vi "加载界面.vi"() -> ()   [LabVIEW 2019]
panel:
  out "错误输出":errorcluster
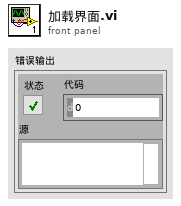
[diagram p1: front panel]
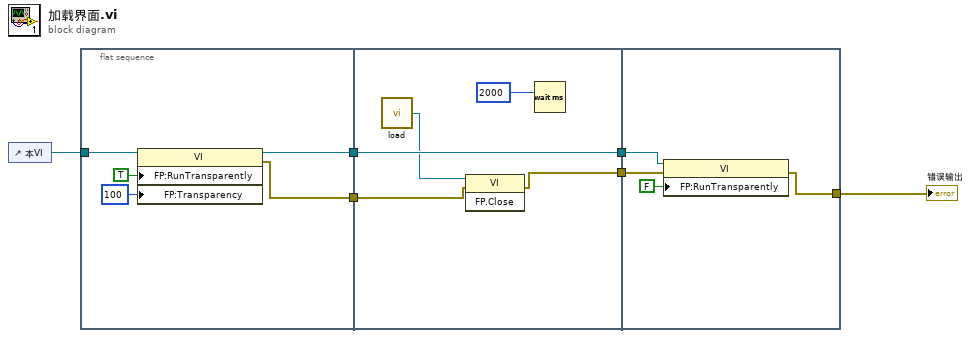
[diagram p0: block diagram]
diagram:
  n1 = control-ref of="本VI"() -> (w6:refnum<vi>)
  n2 = flat-sequence {
    tunnel: w6 -> [w11]
    tunnel: [w8] -> w4
    tunnel: [w7] -> w3
    tunnel: [w15] -> w5
    tunnel: w4 -> [w15]
    tunnel: w3 -> [w14]
    tunnel: [w13] -> w2
    tunnel: w5 -> [w20]
    tunnel: w2 -> [w18]
    tunnel: [w17] -> w1
    frame #0 {
      n3 = property class="VI"(reference=w11, "FP:RunTransparently"=TRUE ("前面板窗口:以透明方式运行VI"), "FP:Transparency"=u8 100 ("前面板窗口:透明度")) -> (reference out=w8:refnum<vi>, error out=w7:errorcluster)  [unwired: 1 in]
    }
    frame #1 {
      n4 = call "load.vi"() -> ("This VI"=w12:refnum<vi>)
      n5 = invoke class="VI" method="FP.Close"(reference=w12, error in=w14) -> (error out=w13:errorcluster)  [unwired: 1 in, 2 out]
      n6 = Wait (ms)(milliseconds to wait=u32 2000 ("等待时间（毫秒）")) -> ()  [unwired: 1 out]
    }
    frame #2 {
      n7 = property class="VI"(reference=w20, error in=w18, "FP:RunTransparently"=FALSE ("前面板窗口:以透明方式运行VI")) -> (error out=w17:errorcluster)  [unwired: 1 out]
    }
  }
  "错误输出" <- w1
